vi "PortionArray.vi"(0 "Width":dbl format="%.2f", 3 "Index":dbl format="%.2f", 4 "Tableau":dbl[](array[numeric]) format="%.2f") -> (1 "Tableau Out":dbl[](array[numeric]) format="%.2f")   [LabVIEW 2009]
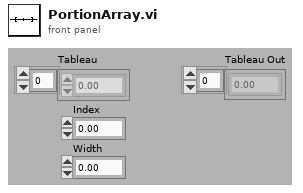
[diagram p1: front panel]
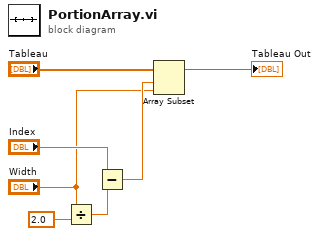
[diagram p0: block diagram]
diagram:
  n1 = Divide(x="Width", y=2.0) -> (x/y=w3:dbl)
  n2 = Subtract(x="Index", y=w3) -> (x-y=w2:dbl)
  n3 = Array Subset(array="Tableau", index=w2, length="Width") -> (→"Tableau Out":dbl[])
